vi "FTW-JSON-SetFlags-Encoding.vi"(0 "JSON":refnum<class "FTW-Container.lvclass">, 5 "Indent Spaces":i32=4, 7 "Escape Unicode":bool=TRUE, 9 "Sort Keys":bool, 11 "error in":errorcluster, 12 "Floating Point Significant Digits":i32=16) -> (4 "JSON out":refnum<class "FTW-Container.lvclass">, 15 "error out":errorcluster)   [LabVIEW 2015]
uses:
  container/FTW-Container.lvclass
panel:
  # "Inputs"
  # "Outputs"
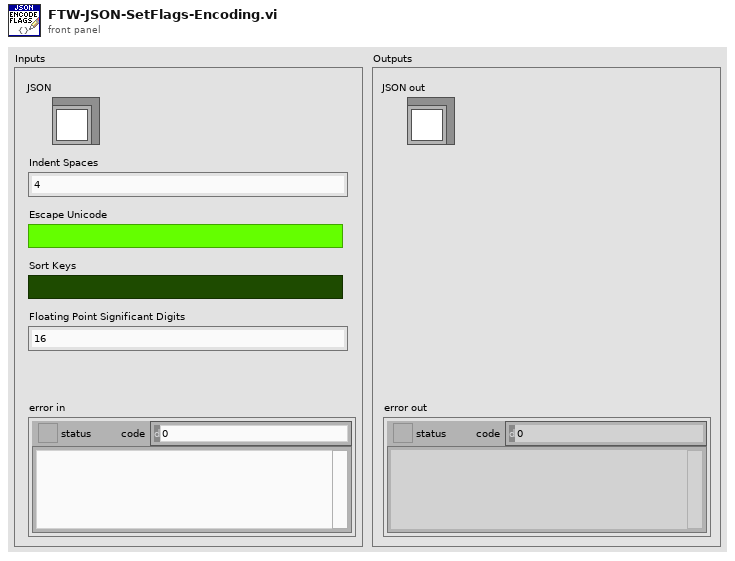
[diagram p1: front panel]
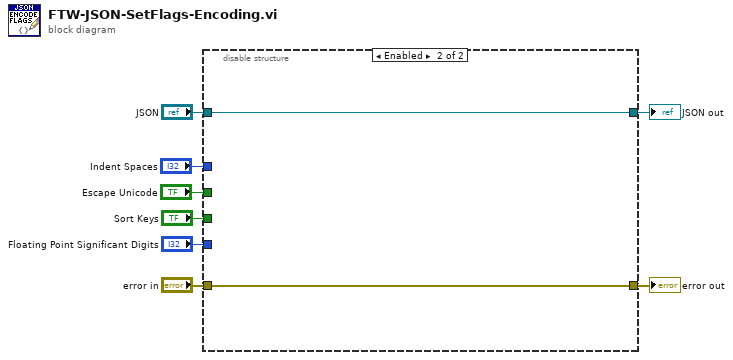
[diagram p0: block diagram]
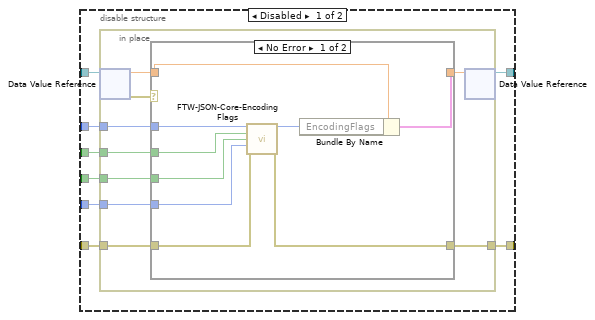
[diagram p2: hidden frame]
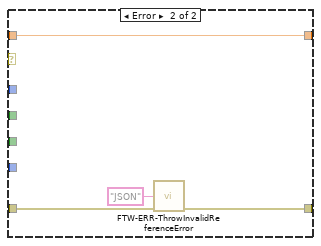
[diagram p3: hidden frame]
diagram:
  n1 = disable-structure shown="Enabled" {
    disable-tunnel: "Indent Spaces" -> [w16 _]
    disable-tunnel: "Escape Unicode" -> [w15 _]
    disable-tunnel: "Sort Keys" -> [w14 _]
    disable-tunnel: "Floating Point Significant Digits" -> [w13 _]
    disable-tunnel: "error in" -> [w12 w39]
    disable-tunnel: [w11 w39] -> w3
    disable-tunnel: "JSON" -> [w10 w40]
    disable-tunnel: [w9 w40] -> w1
    frame Disabled {
      n2 = in-place {
        in-place-border: w16 -> [w25]
        in-place-border: w15 -> [w24]
        in-place-border: w14 -> [w23]
        in-place-border: w13 -> [w22]
        in-place-border: w12 -> [w21]
        in-place-border: [w20] -> w11
        n3 = in-place-dvr #1(w10) -> (w19:dbl, w17:errorcluster)
        n4 = case shown="No Error" w17 {
          tunnel: w25 -> [w34 _]
          tunnel: w24 -> [w33 _]
          tunnel: w23 -> [w32 _]
          tunnel: w22 -> [w31 _]
          tunnel: w21 -> [w29 w36]
          tunnel: [w28 w35] -> w20
          tunnel: w19 -> [w27 w38]
          tunnel: [w26 w38] -> w18
          frame No Error {
            n5 = call "FTW-JSON-Core-EncodingFlags.vi"("Indent Spaces"=w34, "Escape Unicode"=w33, "Sort Keys"=w32, "Floating Point Significant Digits"=w31, "error in"=w29) -> ("Encoding Flags"=w30:i64, "error out"=w28:errorcluster)  [unwired: 9 in]
            n6 = Bundle By Name(cluster=w27, "EncodingFlags"=w30) -> (w26:cluster{})
          }
          frame Error {
            n7 = call "FTW-ERR-ThrowInvalidReferenceError.vi"("Reference Type"="JSON", "error in"=w36) -> ("error out"=w35:errorcluster)  [unwired: 13 in]
          }
        }
        n8 = in-place-dvr #1(w18) -> (w9:refnum<data-value>)  [unwired: 1 out]
      }
    }
    frame Enabled {
    }
  }
  "error out" <- w3
  "JSON out" <- w1
